vi "Basic Backup Test.vi"() -> (0 "error out":errorcluster)   [LabVIEW 2014, in "SQLite3LV Tests.lvlib"]
uses:
  SQLite3LV Tests.lvlib
  SQLite3LV/Cursor Class/property binding/column I32.vi
  SQLite3LV/Cursor Class/property binding/column Text.vi
  SQLite3LV/SQLite3 Class/sqlite3.lvclass
  SQLite3LV/Cursor Class/cursor.lvclass
panel:
  out "progress":u8(slide) scale=0.0..100.0
  out "Array":T1(array[cluster])
  # "This VI will create and write to an in-memory database,\nthen execute a backup to a file-based database.\nIt then reads the values out of the file-based database before deleting it."
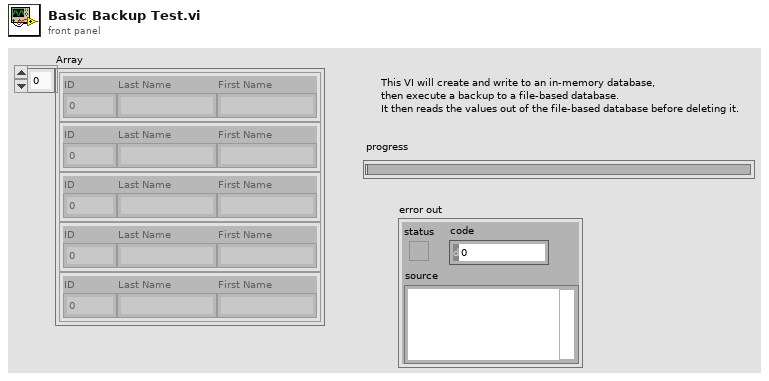
[diagram p1: front panel]
types:
  T1 = cluster{"ID":i32, "Last Name":string, "First Name":string}[]
  T2 = cluster{"property binding:Column I32":i32, "property binding:Column Text":string, "property binding:Column Text":string}
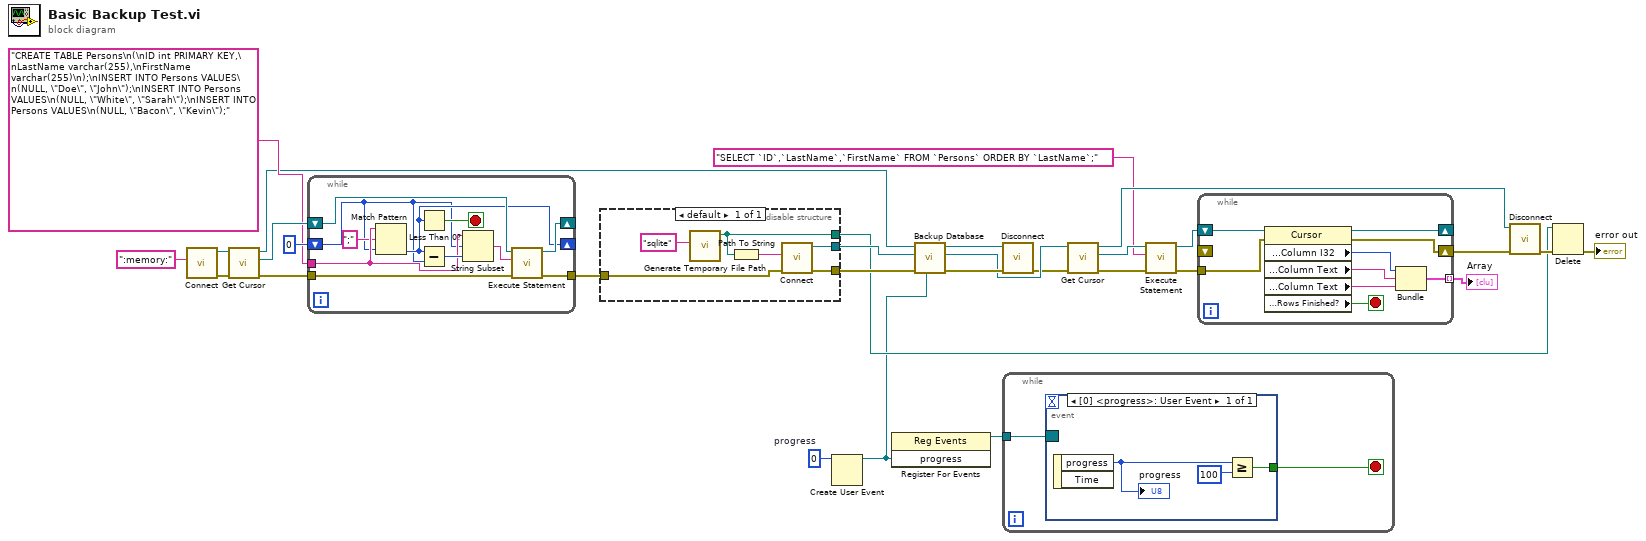
[diagram p0: block diagram]
diagram:
  w3 = u8 0  # progress
  n1 = call "Connect.vi"("path"=":memory:" ("path_utf8")) -> ("error out"=w27:errorcluster, "SQLite3LV Connection out"=w28:refnum<class "sqlite3.lvclass">)  [unwired: 9 in]
  n2 = call "Get Cursor.vi"("error in (no error)"=w27, "SQLite3LV Connection in"=w28) -> ("error out"=w25:errorcluster, "SQLite3LV Cursor"=w26:refnum<class "cursor.lvclass">, "SQLite3LV Connection out"=w22:refnum<class "sqlite3.lvclass">)  [unwired: 7 in]
  n3 = while {
    tunnel: [w38] -> w20
    tunnel: w25 -> [w37]
    shift-right: [w31] -> _
    shift-left: 0 -> [w30]
    tunnel: "CREATE TABLE Persons\n(\nID int PRIMARY KEY,\nLastName varchar(255),\nFirstName varchar(255)\n);\nINSERT INTO Persons VALUES\n(NULL, \"Doe\", \"John\");\nINSERT INTO Persons VALUES\n(NULL, \"White\", \"Sarah\");\nINSERT INTO Persons VALUES\n(NULL, \"Bacon\", \"Kevin\");" ("statement") -> [w33]
    shift-right: [w39] -> _
    shift-left: w26 -> [w40]
    stop <- w36 stop-if-true
    n4 = Match Pattern(string=w33, regular expression=";", offset (0)=w30) -> (offset past match=w31:i32)  [unwired: 3 out]
    n5 = Less Than 0?(x=w31) -> (x < 0?=w36:bool)
    n6 = Subtract(x=w31, y=w30) -> (x-y=w35:i32)
    n7 = String Subset(string=w33, offset (0)=w30, length (rest)=w35) -> (substring=w34:string)
    n8 = call "Execute Statement.vi"("error in (no error)"=w37, "SQL statement"=w34, "SQLite3LV Cursor in"=w40) -> ("error out"=w38:errorcluster, "SQLite3LV Cursor out"=w39:refnum<class "cursor.lvclass">)  [unwired: 7 in]
  }
  n9 = disable-structure shown="default" {
    disable-tunnel: [w44] -> w21
    disable-tunnel: w20 -> [w43]
    disable-tunnel: [w42] -> w19
    disable-tunnel: [w41] -> w5
    frame Enabled {
      n10 = call <vilib>:"Generate Temporary File Path.vi"("Temporary File Extension (tmp)"="sqlite") -> ("Unique Temporary File Path"=w41:path)  [unwired: 9 in, 1 out]
      n11 = Path To String(path=w41) -> (string=w45:string)
      n12 = call "Connect.vi"("error in (no error)"=w43, "path"=w45) -> ("error out"=w42:errorcluster, "SQLite3LV Connection out"=w44:refnum<class "sqlite3.lvclass">)  [unwired: 8 in]
    }
  }
  n13 = Create User Event(user event datatype=w3) -> (user event=w1:refnum<user-event>)  [unwired: 1 in, 1 out]
  n14 = register-events(w1) -> (reference out=w2:refnum<event-registration>)  [unwired: 2 in, 1 out]
  n15 = call "Backup Database.vi"("progress event"=w1, "error in (no error)"=w19, "SQLite3LV Connection dst"=w21, "SQLite3LV Connection src"=w22) -> ("error out"=w17:errorcluster, "SQLite3LV Connection out (dst)"=w16:refnum<class "sqlite3.lvclass">, "SQLite3LV Connection out (src)"=w18:refnum<class "sqlite3.lvclass">)  [unwired: 5 in]
  n16 = call "Disconnect.vi"("error in (no error)"=w17, "SQLite3LV Connection in"=w18) -> ("error out"=w15:errorcluster)  [unwired: 9 in]
  n17 = while {
    tunnel: w2 -> [w48]
    stop <- w47 stop-if-true
    n18 = event shown="[0] <progress>: User Event" {
      selector: w48 -> [_]
      dyn-events: _ -> [_]
      timeout: _ -> [_]
      tunnel: [w50] -> w47
      event User Event {
        n19 = event-data() -> ("progress"=w49:u8)  [unwired: 1 in, 1 out]
        "progress" <- w49
        n20 = Greater Or Equal?(x=w49, y=100) -> (x >= y?=w50:bool)
      }
    }
  }
  n21 = call "Get Cursor.vi"("error in (no error)"=w15, "SQLite3LV Connection in"=w16) -> ("error out"=w12:errorcluster, "SQLite3LV Cursor"=w13:refnum<class "cursor.lvclass">, "SQLite3LV Connection out"=w14:refnum<class "sqlite3.lvclass">)  [unwired: 7 in]
  n22 = call "Execute Statement.vi"("error in (no error)"=w12, "SQL statement"="SELECT `ID`,`LastName`,`FirstName` FROM `Persons` ORDER BY `LastName`;", "SQLite3LV Cursor in"=w13) -> ("error out"=w9:errorcluster, "SQLite3LV Cursor out"=w10:refnum<class "cursor.lvclass">)  [unwired: 7 in]
  n23 = while {
    tunnel: w9 -> [w59]
    shift-right: [w58] -> _
    shift-left: w10 -> [w60]
    shift-right: [w57] -> w7
    shift-left: _ -> [_]
    tunnel: [w52] -> w8 mode=indexing
    stop <- w56 stop-if-true
    n24 = property class="Cursor"(reference=w60, error in=w59) -> (reference out=w58:refnum<class "cursor.lvclass">, error out=w57:errorcluster, "property binding:Column I32"=w55:i32, "property binding:Column Text"=w54:string, "property binding:Column Text"=w53:string, "property binding:Rows Finished?"=w56:bool)
    n25 = Bundle("property binding:Column I32"=w55, "property binding:Column Text"=w54, "property binding:Column Text"=w53) -> (w52:T2)  [unwired: 1 in]
  }
  "Array" <- w8
  n26 = call "Disconnect.vi"("error in (no error)"=w7, "SQLite3LV Connection in"=w14) -> ("error out"=w6:errorcluster)  [unwired: 9 in]
  n27 = Delete(path (use dialog)=w5, error in=w6) -> (error out=→"error out":errorcluster)  [unwired: 3 in, 2 out]
